vi "procesSiMAGE.vi"(0 "Cam Cluster out":T2={"incident ANGLE COMPENSATION"=[], "dp/B [MeV/C/B]"=[], "charge compensation"=[], "Momentum [MeV/C]"=[], "energyDependence Input"=[], "pixel angle (y)"=[], "dp [MeV/C/] "=[], "angle 2Dfor spectrumj"=[], "dp [MeV/C] 2D"=[], "charge compensation 2D"=[], "Screen&Camera 2"={"Screen Orientation"="Regular", "Screen angle"="Flat", "Lens"=enum."FL1-f8x08", "Calibration (mm/pix)"=1.0}, "ROI info"={"npix-X"=0, "npix-Y"=0, "Left [pix]"=0.0, "Top [pix]"=0.0}, "Y 2D full angle"=[], "calib pixel"={"y1(pixel)"=[], "y2(pixel)"=[], "dp/B [MeV/C/B] (pixel)"=[], "energyDependence Input(pixel)"=[], "bending angle [deg](pixel)"=[], "total path(pixel)"=[], "pixel angle (y)(pixel)"=[], "energy dependence (pixel)"=[], "charge compensation (pixel)"=[], "Momentum [MeV/C](pixel)"=[], "angular compensation(pixel)"=[]}, "2D"={"dp"=[], "chargeCompensation"=[], "angle"=[], "Momentum"=[]}, "UserROI"={"Width"=0.0, "Hight"=0.0, "OffsetX"=0.0, "OffsetY"=0.0}, "final"={"X"=[], "xi"=[], "delta momentum"=0.0, "Y"=[], "yi"=[], "angle (Y)"=[], "delta angle"=0.0, "scale delta angle"=0.0, "intraX"=0.0, "intraY"=0.0, "mask"=[]}, "B[T]"=0.0, "index"=0.0}, 1 "Image":T1, 2 "empty image":bool, 12 "B [T]":dbl) -> (4 "Cam Cluster out 2":T2={"incident ANGLE COMPENSATION"=[], "dp/B [MeV/C/B]"=[], "charge compensation"=[], "Momentum [MeV/C]"=[], "energyDependence Input"=[], "pixel angle (y)"=[], "dp [MeV/C/] "=[], "angle 2Dfor spectrumj"=[], "dp [MeV/C] 2D"=[], "charge compensation 2D"=[], "Screen&Camera 2"={"Screen Orientation"="Regular", "Screen angle"="Flat", "Lens"=enum."FL1-f8x08", "Calibration (mm/pix)"=1.0}, "ROI info"={"npix-X"=0, "npix-Y"=0, "Left [pix]"=0.0, "Top [pix]"=0.0}, "Y 2D full angle"=[], "calib pixel"={"y1(pixel)"=[], "y2(pixel)"=[], "dp/B [MeV/C/B] (pixel)"=[], "energyDependence Input(pixel)"=[], "bending angle [deg](pixel)"=[], "total path(pixel)"=[], "pixel angle (y)(pixel)"=[], "energy dependence (pixel)"=[], "charge compensation (pixel)"=[], "Momentum [MeV/C](pixel)"=[], "angular compensation(pixel)"=[]}, "2D"={"dp"=[], "chargeCompensation"=[], "angle"=[], "Momentum"=[]}, "UserROI"={"Width"=0.0, "Hight"=0.0, "OffsetX"=0.0, "OffsetY"=0.0}, "final"={"X"=[], "xi"=[], "delta momentum"=0.0, "Y"=[], "yi"=[], "angle (Y)"=[], "delta angle"=0.0, "scale delta angle"=0.0, "intraX"=0.0, "intraY"=0.0, "mask"=[]}, "B[T]"=0.0, "index"=0.0}, 6 "Sum Y":cluster{"Ramp Pattern":dbl[], dbl[]}, 8 "spec cluster":cluster{"dp [MeV/C]":dbl[], dbl[]}(graph), 10 "z":dbl[][](array[numeric]), 14 "time":u32)   [LabVIEW 2013]
uses:
  calib_Sub_Typdef.ctl
  SubVis/ScreenCam2_TypDEf.ctl
  SubVis/CamAndObj_TypDEf.ctl
  SubVis/ROIInfo_TypDef.ctl
  SubVis/calibPixel.ctl
  SubVis/2DTypDef.ctl
  SubVis/CamRoiTypDef.ctl
  SubVis/finalCalibTypdef.ctl
  <vilib>/vision/Image Controls.llb/IMAQ Image.ctl
panel:
  out "time 2":u32
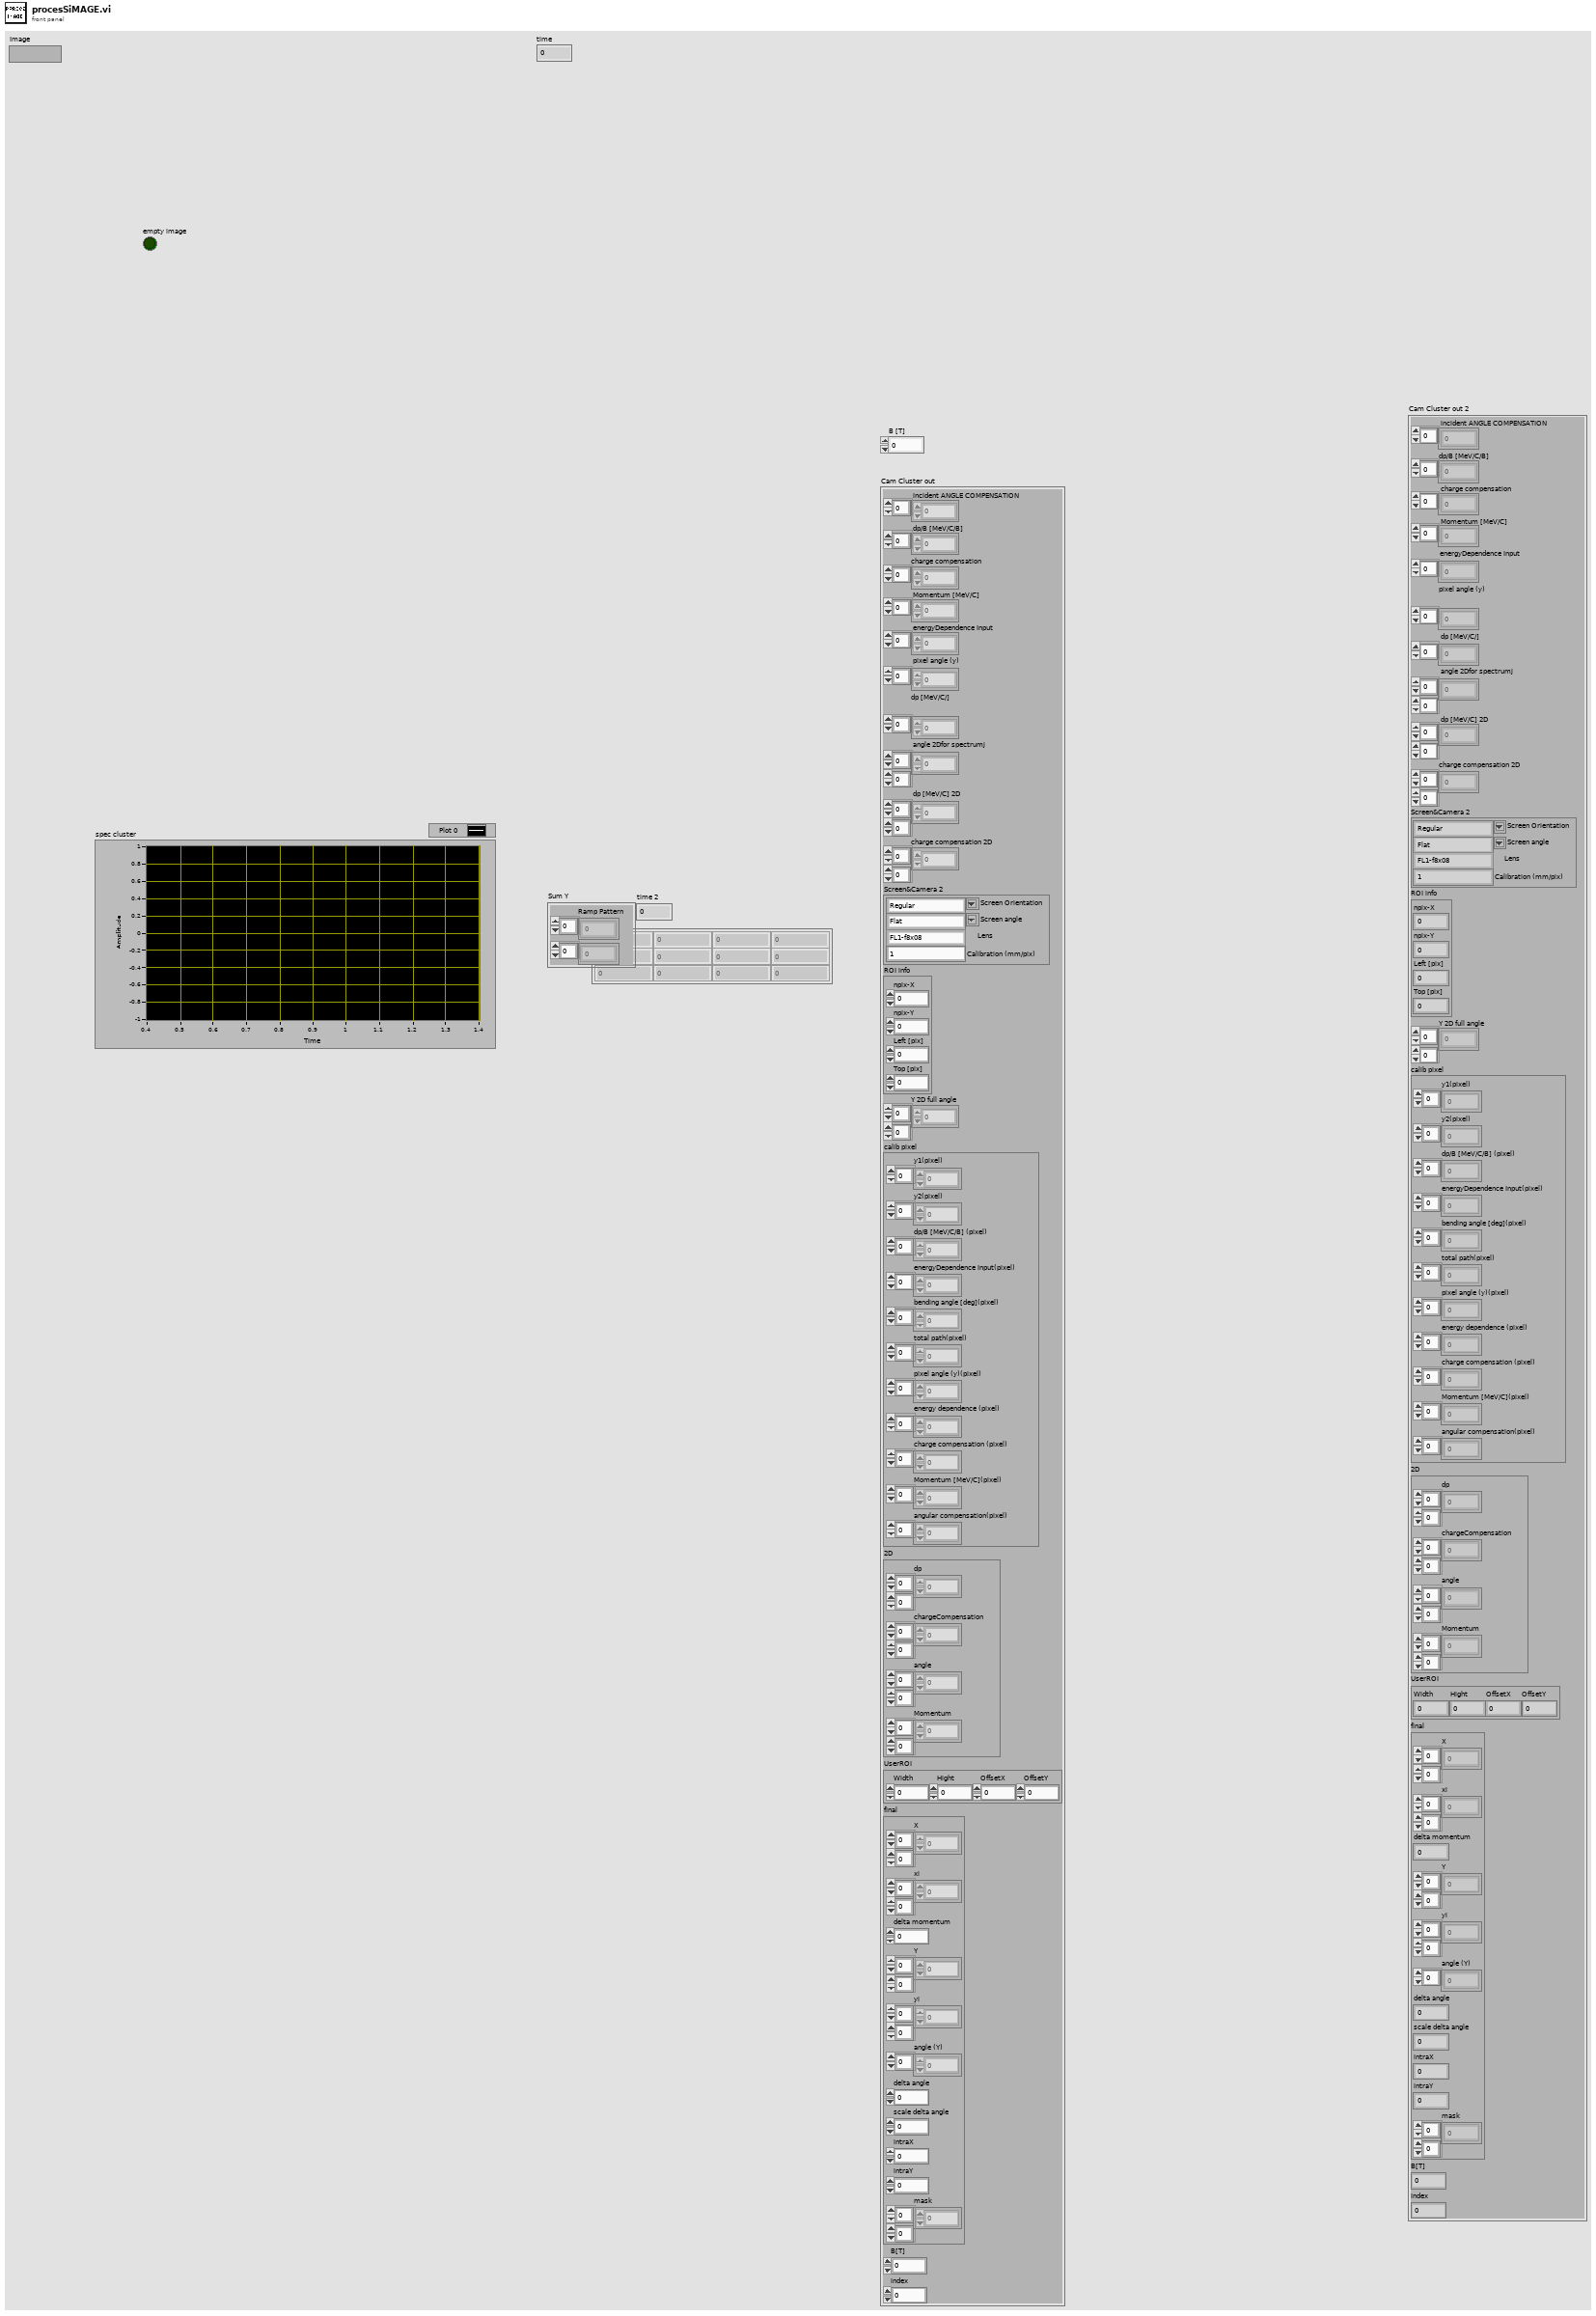
[diagram p1: front panel]
types:
  T1 = typedef "IMAQ Image.ctl" = refnum<image>
  T2 = typedef "calib_Sub_Typdef.ctl" = cluster{"incident ANGLE COMPENSATION":dbl[], "dp/B [MeV/C/B]":dbl[], "charge compensation":dbl[], "Momentum [MeV/C]":dbl[], "energyDependence Input":dbl[], "pixel angle (y)":dbl[], "dp [MeV/C/] ":dbl[], "angle 2Dfor spectrumj":dbl[][], "dp [MeV/C] 2D":dbl[][], "charge compensation 2D":dbl[][], "Screen&Camera 2":T3, "ROI info":T5, "Y 2D full angle":dbl[][], "calib pixel":T6, "2D":T7, "UserROI":T8, "final":T9, "B[T]":dbl, "index":dbl}
  T3 = typedef "ScreenCam2_TypDEf.ctl" = cluster{"Screen Orientation":string, "Screen angle":string, "Lens":T4, "Calibration (mm/pix)":dbl}
  T4 = typedef "CamAndObj_TypDEf.ctl" = enum16{"FL1-f8x08", "FL1-f8x06", "FL1-f8", "ch300-f50", "FL2G-f8", "FL3M14-f8", "FL3M14-f8x08", "FL3M14-f8x08(2x2)"}
  T5 = typedef "ROIInfo_TypDef.ctl" = cluster{"npix-X":i32, "npix-Y":i32, "Left [pix]":dbl, "Top [pix]":dbl}
  T6 = typedef "calibPixel.ctl" = cluster{"y1(pixel)":dbl[], "y2(pixel)":dbl[], "dp/B [MeV/C/B] (pixel)":dbl[], "energyDependence Input(pixel)":dbl[], "bending angle [deg](pixel)":dbl[], "total path(pixel)":dbl[], "pixel angle (y)(pixel)":dbl[], "energy dependence (pixel)":dbl[], "charge compensation (pixel)":dbl[], "Momentum [MeV/C](pixel)":dbl[], "angular compensation(pixel)":dbl[]}
  T7 = typedef "2DTypDef.ctl" = cluster{"dp":dbl[][], "chargeCompensation":dbl[][], "angle":dbl[][], "Momentum":dbl[][]}
  T8 = typedef "CamRoiTypDef.ctl" = cluster{"Width":dbl, "Hight":dbl, "OffsetX":dbl, "OffsetY":dbl}
  T9 = typedef "finalCalibTypdef.ctl" = cluster{"X":dbl[][], "xi":dbl[][], "delta momentum":dbl, "Y":dbl[][], "yi":dbl[][], "angle (Y)":dbl[], "delta angle":dbl, "scale delta angle":dbl, "intraX":dbl, "intraY":dbl, "mask":dbl[][]}
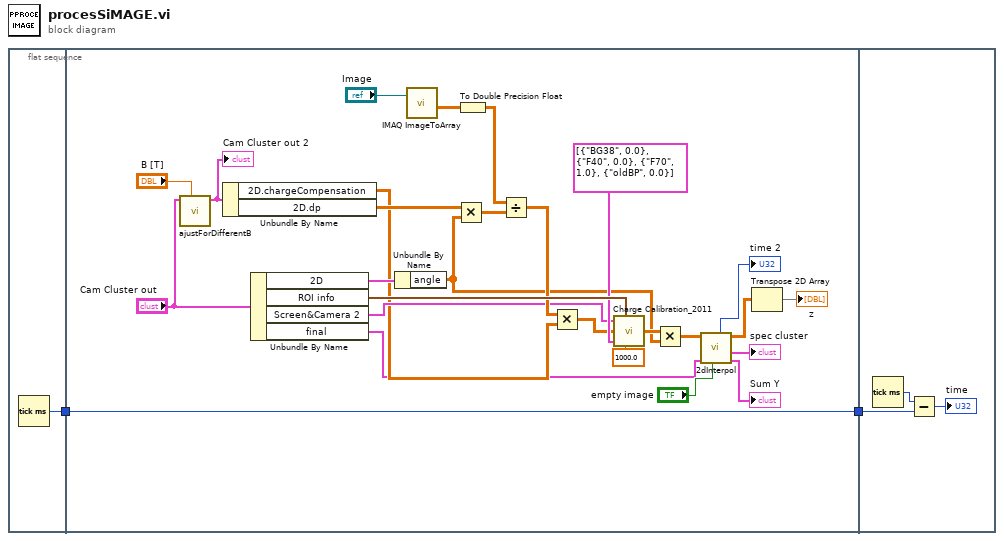
[diagram p0: block diagram]
diagram:
  n1 = flat-sequence {
    tunnel: [w3] -> w1
    tunnel: [w29] -> w2
    tunnel: w1 -> [w29]
    tunnel: w2 -> [w32]
    frame #0 {
      n2 = Tick Count (ms)() -> (millisecond timer value=w3:u32)
    }
    frame #1 {
      n3 = call "ajustForDifferentB.vi"("B [T]"="B [T]", "Cam Cluster out in"="Cam Cluster out") -> ("Cam Cluster out out"=w6:T2)  [unwired: 8 in, 1 out]
      "Cam Cluster out 2" <- w6
      n4 = Unbundle By Name(w6) -> ("2D.chargeCompensation"=w11:dbl[][], "2D.dp"=w12:dbl[][])
      n5 = Unbundle By Name("Cam Cluster out") -> ("2D"=w13:T7, "ROI info"=w28:T5, "Screen&Camera 2"=w15:T3, "final"=w5:T9)
      n6 = Unbundle By Name(w13) -> ("angle"=w14:dbl[][])
      n7 = call "IMAQ ImageToArray"("Image"="Image") -> ("Image Pixels (Float)"=w19:sgl[][])  [unwired: 3 in, 4 out]
      n8 = Multiply(x=w12, y=w14) -> (x*y=w27:dbl[][])
      n9 = To Double Precision Float(number=w19) -> (double precision float=w18:dbl[][])
      n10 = Divide(x=w18, y=w27) -> (x/y=w24:dbl[][])
      n11 = Multiply(x=w24, y=w11) -> (x*y=w17:dbl[][])
      n12 = call "Charge Calibration_2011.vi"("Screen&Camera 2"=w15, "ROI infos"=w28, "Image (Counts)"=w17, "Filters"=cluster{"Name":string, "#Filters":dbl}[] [{"Name"="BG38", "#Filters"=0.0}, {"Name"="F40", "#Filters"=0.0}, {"Name"="F70", "#Filters"=1.0}, {"Name"="oldBP", "#Filters"=0.0}], "Electron energy (MeV)"=1000.0) -> ("Image (pC)"=w23:dbl[][])  [unwired: 4 in]
      n13 = Multiply(x=w23, y=w14) -> (x*y=w22:dbl[][])
      n14 = call "2dInterpol.vi"("empty image"="empty image", "final"=w5, "Z"=w22) -> ("Sum Y"=→"Sum Y":cluster{"Ramp Pattern":dbl[], dbl[]}, "spec cluster 2"=→"spec cluster":cluster{"Momentum [MeV/C]":dbl[], dbl[]}, "charge density"=w4:dbl[][], "time: 2Dinter"=→"time 2":u32)  [unwired: 5 in]
      n15 = Transpose 2D Array(2D array=w4) -> (transposed array=→"z":dbl[][])
    }
    frame #2 {
      n16 = Tick Count (ms)() -> (millisecond timer value=w33:u32)
      n17 = Subtract(x=w33, y=w32) -> (x-y=→"time":u32)
    }
  }
